vi "Vision Processing.vi"(4 "error in (no error)":errorcluster, 7 "Image Size":T3=enum."320x240") -> ()   [LabVIEW 2014]
doc: "This VI runs in parallel to other tasks. It gets images from the camera, processes them for color or shape and use that information to affect robot behavior."
uses:
  <vilib>/Rock Robotics/WPI/Camera/WPI_CameraImageSize.ctl
  <vilib>/Rock Robotics/WPI/Camera/WPI_CameraWhite Balance Values.ctl
  <vilib>/Rock Robotics/WPI/Camera/WPI_CameraExposure Values.ctl
  <vilib>/Rock Robotics/WPI/Camera/WPI_CameraFrameRate.ctl
  Robot Global Data.vi
  <vilib>/vision/NI_Vision_Development_Module.lvlib
panel:
  out "Original":T1(plugin-control)
  out "Masked":T1(plugin-control)
  out "Particle Reports (Pixels)":T2(array[cluster]) {"Orientation" format="%.2f"; "Dimensions"."Height" format="%.2f"; "Dimensions"."Width" format="%.2f"; "Center of Mass"."Y" format="%.2f"; "Center of Mass"."X" format="%.2f"; "Bounding Rect"."Bottom" format="%.2f"; "Bounding Rect"."Right" format="%.2f"; "Bounding Rect"."Top" format="%.2f"; "Bounding Rect"."Left" format="%.2f"; "Number of Holes" format="%.2f"; "Area" format="%.2f"}
  out "Particle Reports (Real-World)":T2(array[cluster]) {"Orientation" format="%.2f"; "Dimensions"."Height" format="%.2f"; "Dimensions"."Width" format="%.2f"; "Center of Mass"."Y" format="%.2f"; "Center of Mass"."X" format="%.2f"; "Bounding Rect"."Bottom" format="%.2f"; "Bounding Rect"."Right" format="%.2f"; "Bounding Rect"."Top" format="%.2f"; "Bounding Rect"."Left" format="%.2f"; "Number of Holes" format="%.2f"; "Area" format="%.2f"}
  out "Equalized":T1(plugin-control)
  in  "Red or Hue Range":cluster{"Lower value":i32, "Upper value":i32}={"Lower value"=100, "Upper value"=255}
  in  "Green or Sat Range":cluster{"Lower value":i32, "Upper value":i32}={"Lower value"=100, "Upper value"=175}
  in  "Blue or Luma or Val or Inten Range":cluster{"Lower value":i32, "Upper value":i32}={"Lower value"=0, "Upper value"=80}
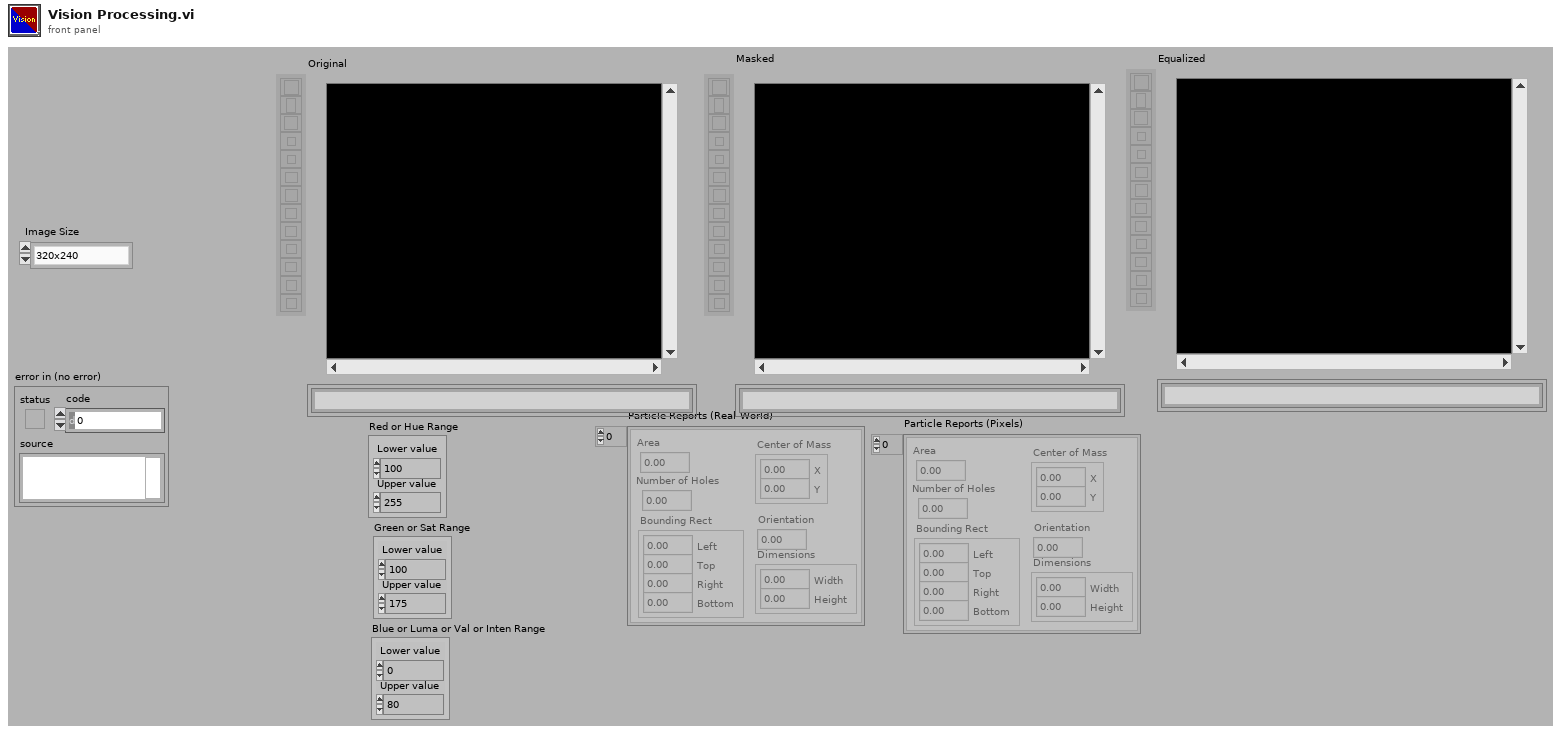
[diagram p1: front panel]
types:
  T1 = typedef "IMAQ Image.ctl" = refnum<image>
  T2 = cluster{"Area":dbl, "Number of Holes":dbl, "Bounding Rect":cluster{"Left":dbl, "Top":dbl, "Right":dbl, "Bottom":dbl}, "Center of Mass":cluster{"X":dbl, "Y":dbl}, "Orientation":dbl, "Dimensions":cluster{"Width":dbl, "Height":dbl}}[]
  T3 = typedef "WPI_CameraImageSize.ctl" = enum16{"640x480", "320x240", "160x120", "Custom"}
  T4 = typedef "Image Type" = u32
  T5 = typedef "WPI_CameraFrameRate.ctl" = u32
  T6 = typedef "WPI_CameraExposure Values.ctl" = enum16{"Auto", "Flicker-free 50 Hz", "Flicker-free 60 Hz", "Hold current", "Custom"}
  T7 = typedef "WPI_CameraWhite Balance Values.ctl" = enum16{"Auto", "Fixed indoor", "Fixed outdoor 1", "Fixed outdoor 2", "Fixed fluorescent 1", "Fixed fluorescent 2", "Hold current", "Custom"}
  T8 = typedef "WPI_CameraDevRef.ctl" = cluster{"Camera Address":string, "CameraStatus":errorcluster}
  T9 = cluster{"Area":dbl, "Number of Holes":dbl, "Bounding Rect":cluster{"Left":dbl, "Top":dbl, "Right":dbl, "Bottom":dbl}, "Center of Mass":cluster{"X":dbl, "Y":dbl}, "Orientation":dbl, "Dimensions":cluster{"Width":dbl, "Height":dbl}}
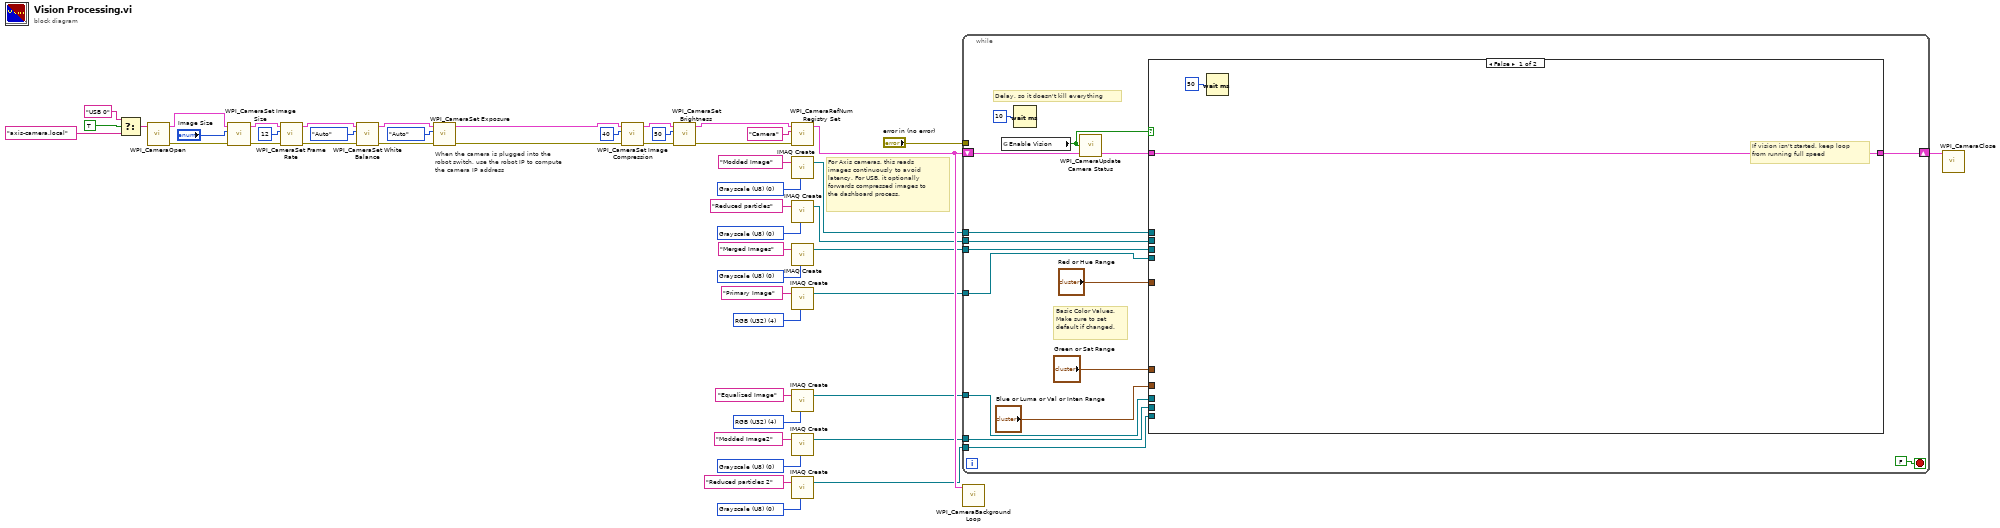
[diagram p0: block diagram]
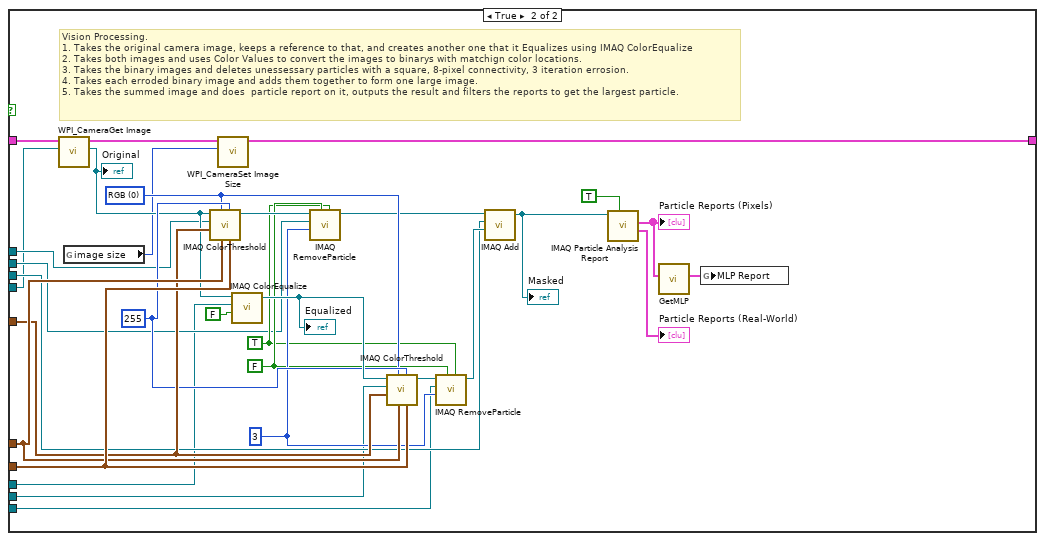
[diagram p2: hidden frame]
diagram:
  w11 = T4 0 items=["Grayscale (U8)", "Grayscale (I16)", "Grayscale (SGL)", "Complex (CSG)", "RGB (U32)", "HSL (U32)", "RGB (U64)"] ("Image Type")
  w13 = T4 0 items=["Grayscale (U8)", "Grayscale (I16)", "Grayscale (SGL)", "Complex (CSG)", "RGB (U32)", "HSL (U32)", "RGB (U64)"] ("Image Type")
  w15 = T4 0 items=["Grayscale (U8)", "Grayscale (I16)", "Grayscale (SGL)", "Complex (CSG)", "RGB (U32)", "HSL (U32)", "RGB (U64)"] ("Image Type")
  w17 = T4 0 items=["Grayscale (U8)", "Grayscale (I16)", "Grayscale (SGL)", "Complex (CSG)", "RGB (U32)", "HSL (U32)", "RGB (U64)"] ("Image Type")
  w19 = T4 4 items=["Grayscale (U8)", "Grayscale (I16)", "Grayscale (SGL)", "Complex (CSG)", "RGB (U32)", "HSL (U32)", "RGB (U64)"] ("Image Type")
  w21 = T4 0 items=["Grayscale (U8)", "Grayscale (I16)", "Grayscale (SGL)", "Complex (CSG)", "RGB (U32)", "HSL (U32)", "RGB (U64)"] ("Image Type")
  w23 = T4 4 items=["Grayscale (U8)", "Grayscale (I16)", "Grayscale (SGL)", "Complex (CSG)", "RGB (U32)", "HSL (U32)", "RGB (U64)"] ("Image Type")
  # "When the camera is plugged into the\nrobot switch, use the robot IP to compute\nthe camera IP address"
  # "For Axis cameras, this reads\nimages continuously to avoid\nlatency. For USB, it optionally\nforwards compressed images to\nthe dashboard process."
  n1 = Select(t="USB 0" ("format string"), s=TRUE ("dot notation? (F)"), f="axis-camera.local" ("format string")) -> (s? t:f=w26:string)
  n2 = call <vilib>:"WPI_CameraOpen.vi"("Camera Address"=w26) -> ("error out"=w40:errorcluster, "CameraDevRef"=w41:T8)  [unwired: 1 in, 8 out]
  n3 = call <vilib>:"WPI_CameraSet Image Size.vi"("error in (no error)"=w40, "Image Size"="Image Size", "CameraDevRef"=w41) -> ("error out"=w39:errorcluster, "CameraDevRef Out"=w42:T8)  [unwired: 1 in, 6 out]
  n4 = call <vilib>:"WPI_CameraSet Frame Rate.vi"("error in (no error)"=w39, "Frame Rate (fps)"=T5 12, "CameraDevRef"=w42) -> ("error out"=w38:errorcluster, "CameraDevRef Out"=w44:T8)  [unwired: 7 out]
  n5 = call <vilib>:"WPI_CameraSet White Balance.vi"("error in (no error)"=w38, "White Balance"=WPI_CameraWhite_Balance_Values."Auto", "CameraDevRef"=w44) -> ("error out"=w37:errorcluster, "CameraDevRef Out"=w43:T8)  [unwired: 1 in, 6 out]
  n6 = call <vilib>:"WPI_CameraSet Exposure.vi"("error in (no error)"=w37, "Exposure"=WPI_CameraExposure_Values."Auto", "CameraDevRef"=w43) -> ("error out"=w36:errorcluster, "CameraDevRef Out"=w46:T8)  [unwired: 1 in, 6 out]
  n7 = call <vilib>:"WPI_CameraSet Image Compression.vi"("error in (no error)"=w36, "Compression"=40, "CameraDevRef"=w46) -> ("error out"=w35:errorcluster, "CameraDevRef Out"=w45:T8)  [unwired: 7 out]
  n8 = call <vilib>:"WPI_CameraSet Brightness.vi"("error in (no error)"=w35, "Brightness"=50, "CameraDevRef"=w45) -> ("error out"=w33:errorcluster, "CameraDevRef Out"=w34:T8)  [unwired: 7 out]
  n9 = call <vilib>:"WPI_CameraRefNum Registry Set.vi"("error in (no error)"=w33, "refnum name"="Camera", "CameraDevRef"=w34) -> ("CameraDevRef"=w24:T8)  [unwired: 8 out]
  n10 = call "IMAQ Create"("Image Name"="Modded Image", "Image Type"=w21) -> ("New Image"=w5:T1)  [unwired: 2 in, 2 out]
  n11 = call "IMAQ Create"("Image Name"="Reduced particles", "Image Type"=w17) -> ("New Image"=w4:T1)  [unwired: 2 in, 2 out]
  n12 = call "IMAQ Create"("Image Name"="Merged Images", "Image Type"=w11) -> ("New Image"=w8:T1)  [unwired: 2 in, 2 out]
  n13 = call "IMAQ Create"("Image Name"="Primary Image", "Image Type"=w23) -> ("New Image"=w3:T1)  [unwired: 2 in, 2 out]
  n14 = call "IMAQ Create"("Image Name"="Equalized Image", "Image Type"=w19) -> ("New Image"=w2:T1)  [unwired: 2 in, 2 out]
  n15 = call "IMAQ Create"("Image Name"="Modded Image2", "Image Type"=w13) -> ("New Image"=w6:T1)  [unwired: 2 in, 2 out]
  n16 = call "IMAQ Create"("Image Name"="Reduced particles 2", "Image Type"=w15) -> ("New Image"=w7:T1)  [unwired: 2 in, 2 out]
  n17 = while {
    shift-right: [w64] -> w1
    shift-left: w24 -> [w63]
    tunnel: "error in (no error)" -> [_]
    tunnel: w8 -> [w57]
    tunnel: w7 -> [w56]
    tunnel: w6 -> [w55]
    tunnel: w5 -> [w54]
    tunnel: w4 -> [w53]
    tunnel: w3 -> [w52]
    tunnel: w2 -> [w51]
    stop <- FALSE stop-if-true
    # "Basic Color Values.\nMake sure to set\ndefault if changed."
    # "Delay, so it doesn't kill everything"
    n18 = global read "Robot Global Data.vi" "Enable Vision"() -> (w50:bool)
    n19 = Wait (ms)(milliseconds to wait=u32 10) -> ()  [unwired: 1 out]
    n20 = call <vilib>:"WPI_CameraUpdate Camera Status.vi"("CameraDevRef In"=w63, "Enable Vision"=w50) -> ("CameraDevRef Out"=w62:T8)  [unwired: 3 in]
    n21 = case shown="False" w50 {
      tunnel: [w67 w98] -> w64
      tunnel: w62 -> [w67 w97]
      tunnel: "Red or Hue Range" -> [_ w89]
      tunnel: "Green or Sat Range" -> [_ w90]
      tunnel: "Blue or Luma or Val or Inten Range" -> [_ w91]
      tunnel: w57 -> [_ w77]
      tunnel: w56 -> [_ w76]
      tunnel: w55 -> [_ w75]
      tunnel: w54 -> [_ w74]
      tunnel: w53 -> [_ w73]
      tunnel: w52 -> [_ w72]
      tunnel: w51 -> [_ w71]
      frame False {
        # "If vision isn't started, keep loop\nfrom running full speed"
        n22 = Wait (ms)(milliseconds to wait=u32 50) -> ()  [unwired: 1 out]
      }
      frame True {
        w83 = TRUE ("Connectivity 4/8 (8)")
        w84 = FALSE ("Square/Hexa (Square)")
        w85 = 3 ("Number of Erosion")
        w87 = 255 ("Replace Value")
        w86 = u16 0 items=["RGB", "HSL", "HSV", "HSI"] ("Color Mode")
        # "Vision Processing.\n1. Takes the original camera image, keeps a reference to that, and creates another one that it Equalizes using IMAQ ColorEqualize\n2. Takes both images and uses Color Values to convert the images to binarys with matchign color locations.\n3. Takes the binary images and deletes unessessary particles with a square, 8-pixel connectivity, 3 iteration errosion.\n4. Takes each erroded binary image and adds them together to form one large image.\n5. Takes the summed image and does  particle report on it, outputs the result and filters the reports to get the largest particle."
        n23 = call <vilib>:"WPI_CameraGet Image.vi"("Image"=w72, "CameraDevRef"=w97) -> ("Image Out"=w81:T1, "CameraDevRef Out"=w96:T8)  [unwired: 1 in, 7 out]
        "Original" <- w81
        n24 = global read "Robot Global Data.vi" "image size"() -> (w70:T3)
        n25 = call "IMAQ ColorThreshold"("Blue or Luma or Val or Inten Range"=w91, "Replace Value"=w87, "Green or Sat Range"=w90, "Color Mode"=w86, "Red or Hue Range"=w89, "Image Dst"=w74, "Image Src"=w81) -> ("Image Dst Out"=w92:T1)  [unwired: 3 in, 1 out]
        n26 = call <vilib>:"WPI_CameraSet Image Size.vi"("Image Size"=w70, "CameraDevRef"=w96) -> ("CameraDevRef Out"=w98:T8)  [unwired: 2 in, 7 out]
        n27 = call "IMAQ ColorEqualize"("Luma / RGB,HSL (Luma)"=FALSE, "Image Dst"=w71, "Image Src"=w81) -> ("Image Dst Out"=w88:T1)  [unwired: 2 in, 1 out]
        "Equalized" <- w88
        n28 = call "IMAQ RemoveParticle"("Connectivity 4/8 (8)"=w83, "Square/Hexa (Square)"=w84, "Number of Erosion"=w85, "Image Dst"=w73, "Image Src"=w92) -> ("Image Dst Out"=w79:T1)  [unwired: 5 in, 1 out]
        n29 = call "IMAQ ColorThreshold"("Blue or Luma or Val or Inten Range"=w91, "Replace Value"=w87, "Green or Sat Range"=w90, "Color Mode"=w86, "Red or Hue Range"=w89, "Image Dst"=w75, "Image Src"=w88) -> ("Image Dst Out"=w82:T1)  [unwired: 3 in, 1 out]
        n30 = call "IMAQ RemoveParticle"("Connectivity 4/8 (8)"=w83, "Square/Hexa (Square)"=w84, "Number of Erosion"=w85, "Image Dst"=w76, "Image Src"=w82) -> ("Image Dst Out"=w78:T1)  [unwired: 5 in, 1 out]
        n31 = call "IMAQ Add"("Image Src A"=w79, "Image Dst"=w77, "Image Src B"=w78) -> ("Image Dst Out"=w80:T1)  [unwired: 4 in, 1 out]
        "Masked" <- w80
        n32 = call "IMAQ Particle Analysis Report"("Connectivity 4/8 (8)"=TRUE, "Image"=w80) -> ("Particle Reports (Real-World)"=→"Particle Reports (Real-World)":T2, "Particle Reports (Pixels)"=w69:T2)  [unwired: 4 in, 4 out]
        "Particle Reports (Pixels)" <- w69
        n33 = call "GetMLP.vi"("Particle Reports (Pixels)"=w69) -> ("MLP Report"=w68:T9)  [unwired: 10 in]
        n34 = global write "Robot Global Data.vi" "MLP Report"(w68) -> ()
      }
    }
  }
  n35 = call <vilib>:"WPI_CameraBackground Loop.vi"("CameraDevRef"=w24) -> ()  [unwired: 11 in]
  n36 = call <vilib>:"WPI_CameraClose.vi"("CameraDevRef"=w1) -> ()  [unwired: 1 in, 10 out]
